vi "Pixy_COM-RIO.vi"() -> (0 "Height":i32, 1 "Width":i32, 2 "Y":i32, 3 "X":i32, 4 "Read error out":errorcluster)   [LabVIEW 2016]
uses:
  <vilib>/Analysis/baseanly.llb/Mean (DBL).vi
  <vilib>/Instr/_visa.llb/VISA Configure Serial Port (Instr).vi
  Cam Area.vi
  Cam H.vi
  Cam W.vi
  Cam Y.vi
  Cam X.vi
  <vilib>/Analysis/NI_AALBase.lvlib
panel:
  in  "Command 2":string(combo)="go"
  out "Initialization error out":errorcluster
  out "Area":dbl(graph)
  in  "Display buffer size":u16=100 min=1
  out "Data display":string
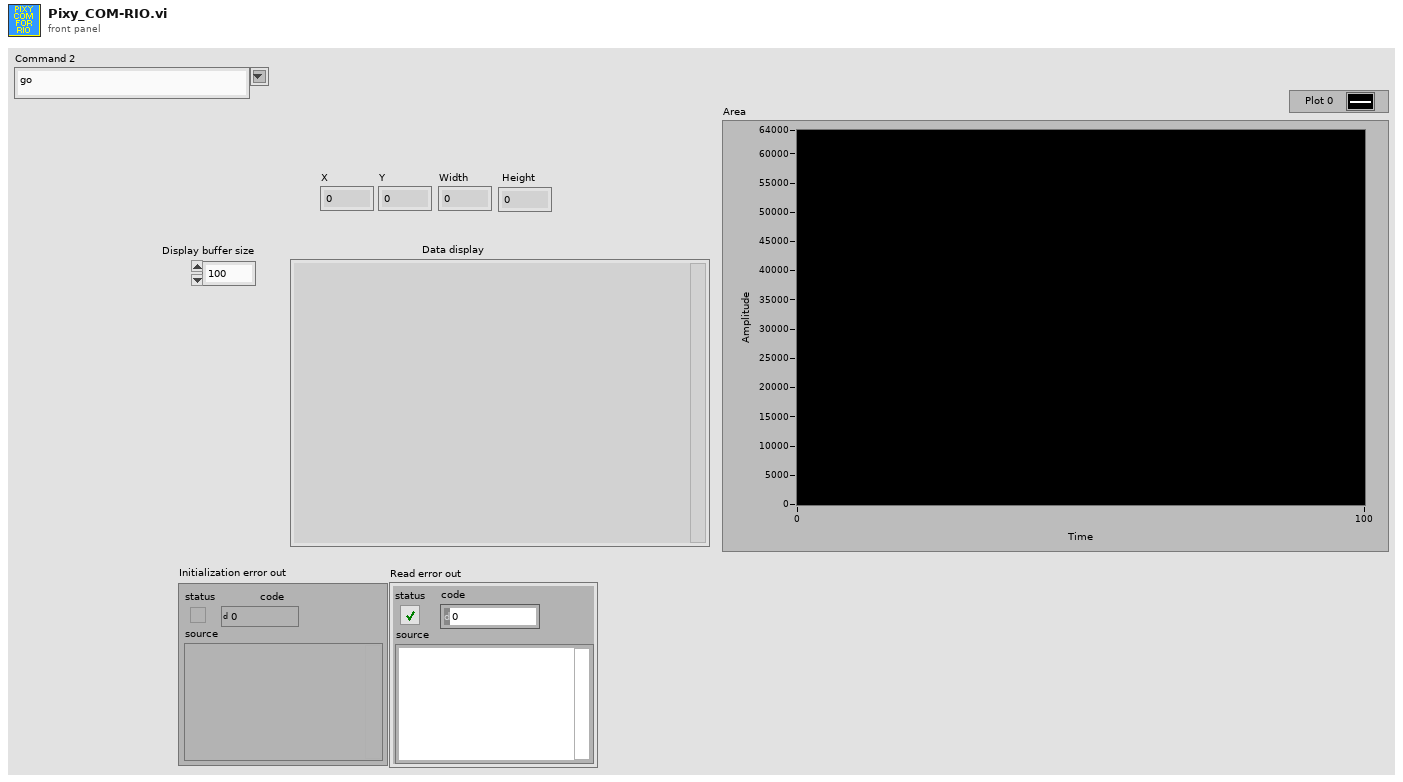
[diagram p1: front panel]
types:
  T1 = cluster{"buffer":string, "X":i32, "Y":i32, "Width":i32, "Height":i32, "Area":dbl}
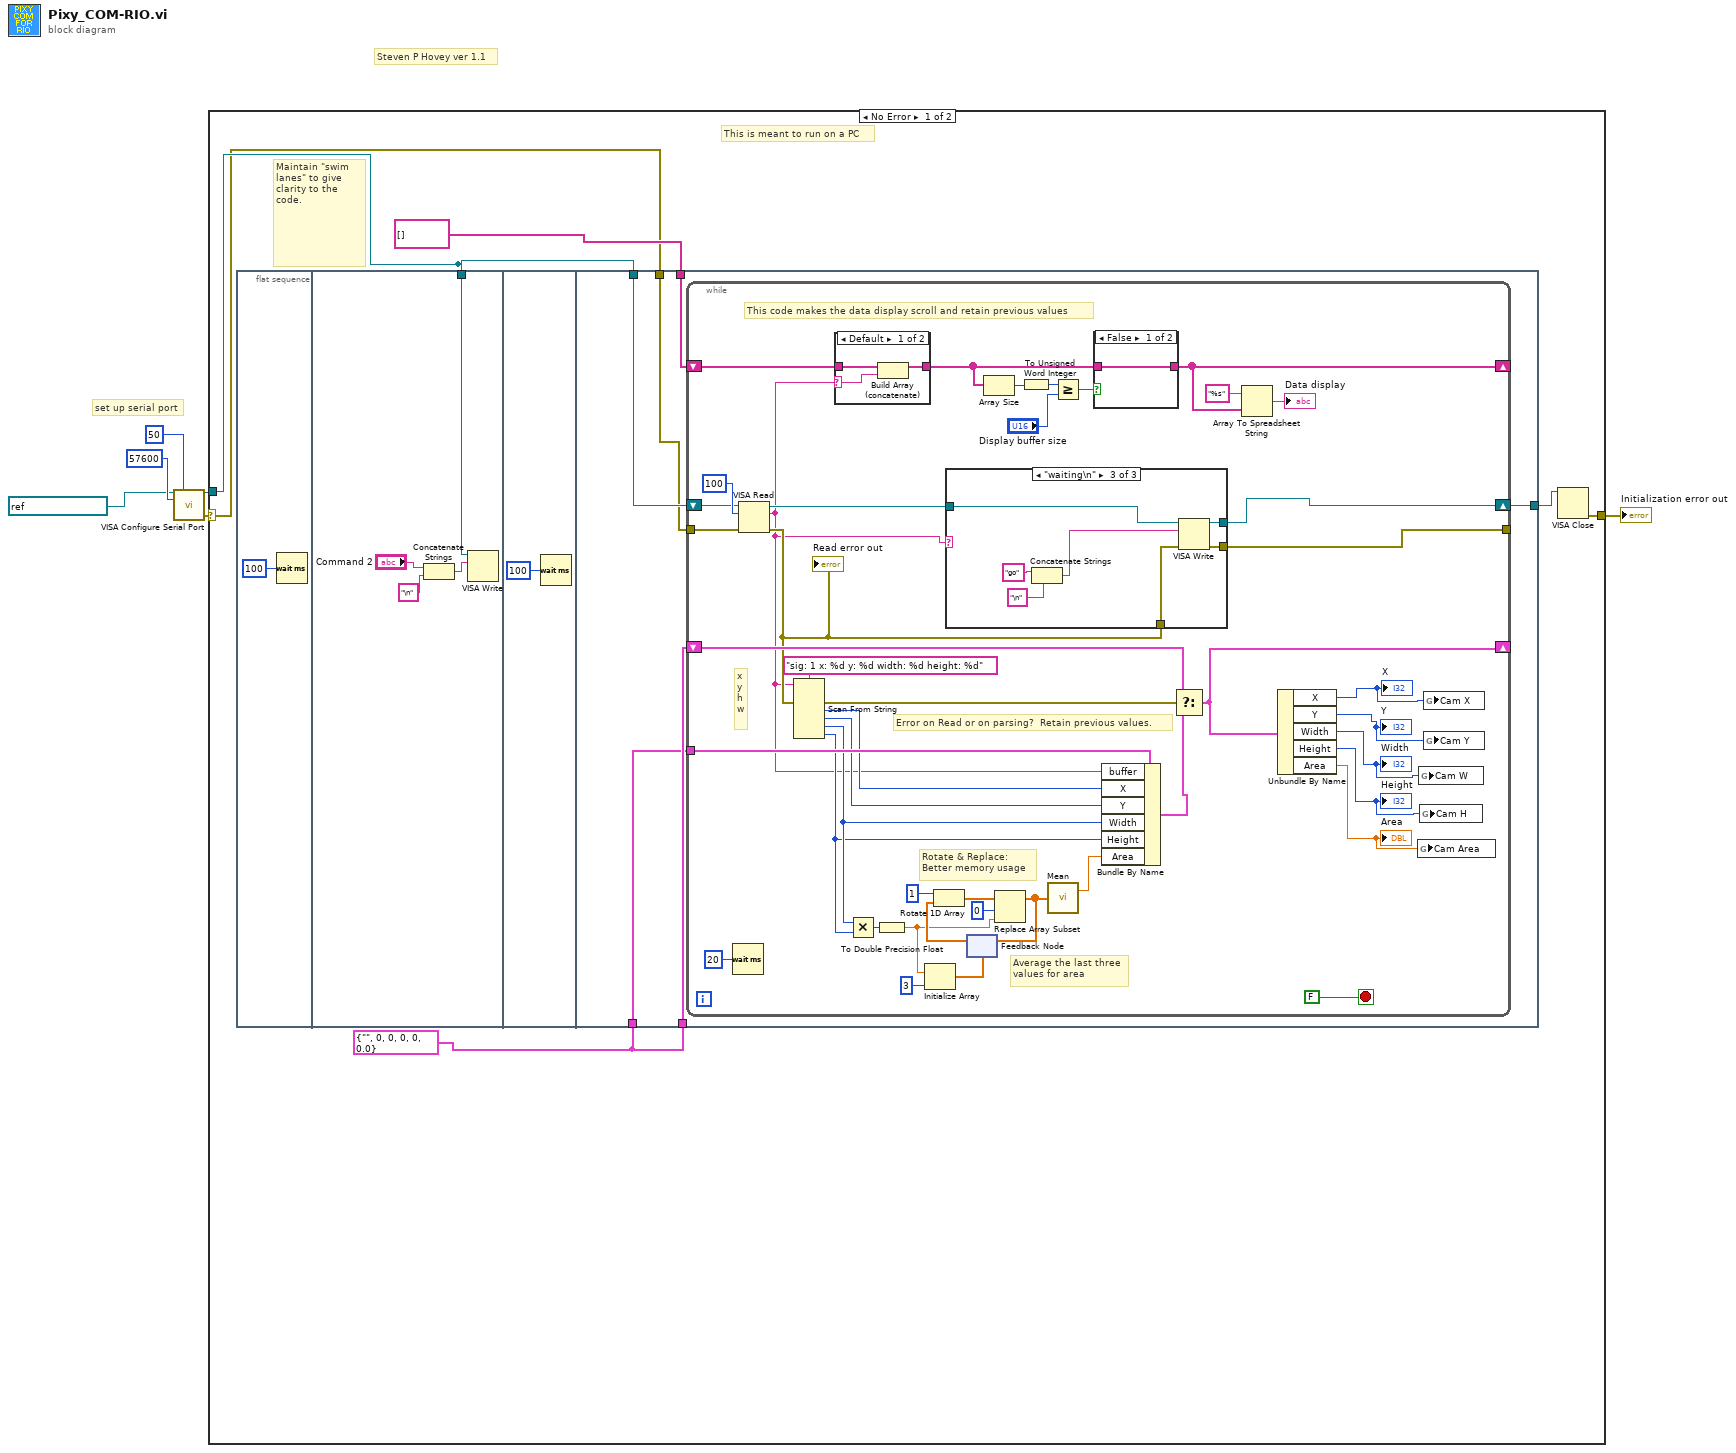
[diagram p0: block diagram]
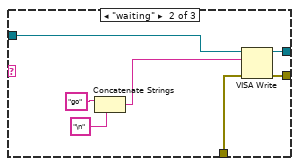
[diagram p3: hidden frame]
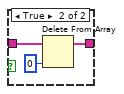
[diagram p5: hidden frame]
diagram:
  # "Steven P Hovey ver 1.1"
  # "set up serial port"
  n1 = call-poly "VISA Configure Serial Port"("VISA resource name"=refnum<visa-resource-name> "ASRL3::INSTR", "timeout (10sec)"=u32 50, "baud rate (9600)"=u32 57600) -> ("VISA resource name out"=w4:refnum<visa-resource-name>, "error out"=w2:errorcluster)  [unwired: 11 in]
  n2 = case shown="No Error" w2 {
    selector: w2 -> [w8 w93]
    tunnel: w4 -> [w9 _]
    tunnel: [w12 w93] -> w3
    frame No Error {
      w10 = T1 {"buffer"="", "X"=0, "Y"=0, "Width"=0, "Height"=0, "Area"=0.0}
      # "Maintain \"swim lanes\" to give clarity to the code."
      # "This is meant to run on a PC"
      n3 = flat-sequence {
        tunnel: w9 -> [w15]
        tunnel: string[] [] -> [w24]
        tunnel: w10 -> [w23]
        tunnel: w10 -> [w22]
        tunnel: w9 -> [w21]
        tunnel: w8 -> [w20]
        tunnel: [w19] -> w7
        frame #0 {
          n4 = Wait (ms)(milliseconds to wait=u32 100) -> ()  [unwired: 1 out]
        }
        frame #1 {
          n5 = Concatenate Strings("Command 2", "\n") -> (w17:string)
          n6 = VISA Write(VISA resource name=w15, write buffer=w17) -> ()  [unwired: 1 in, 3 out]
        }
        frame #2 {
          n7 = Wait (ms)(milliseconds to wait=u32 100) -> ()  [unwired: 1 out]
        }
        frame #3 {
          n8 = while {
            shift-right: [w28] -> w19
            shift-left: w21 -> [w65]
            shift-right: [w44] -> _
            shift-left: w23 -> [w45]
            shift-right: [w38] -> _
            shift-left: w24 -> [w58]
            tunnel: w22 -> [w68]
            tunnel: w20 -> [w37]
            tunnel: [w27] -> _
            stop <- FALSE ("stop") stop-if-true
            # "Error on Read or on parsing?  Retain previous values."
            # "Rotate & Replace:\nBetter memory usage"
            # "Average the last three\nvalues for area"
            # "This code makes the data display scroll and retain previous values"
            # "x\ny\nh\nw"
            n9 = Wait (ms)(milliseconds to wait=u32 20) -> ()  [unwired: 1 out]
            n10 = VISA Read(VISA resource name=w65, byte count=u32 100, error in (no error)=w37) -> (VISA resource name out=w29:refnum<visa-resource-name>, read buffer=w25:string, error out=w26:errorcluster)  [unwired: 1 out]
            "Read error out" <- w26
            n11 = Scan From String(format string="sig: 1 x: %d y: %d width: %d height: %d", input string=w25, error in=w26) -> (error out=w46:errorcluster, output 1=w51:i32, output 2=w50:i32, output 3=w49:i32, output 4=w48:i32)  [unwired: 5 in, 2 out]
            n12 = case shown="Default" w25 {
              selector: w25 -> [w85 _]
              tunnel: w58 -> [w86 w88]
              tunnel: [w87 w88] -> w39
              frame Default {
                n13 = Build Array (concatenate)(w86, w85) -> (w87:string[])
              }
              frame "" {
              }
            }
            n14 = Multiply(x=w49, y=w48) -> (x*y=w47:i32)
            n15 = To Double Precision Float(number=w47) -> (double precision float=w40:dbl)
            n16 = Initialize Array(w40, 3 ("dimension size")) -> (w62:dbl[])
            n17 = case shown="\"waiting\\n\"" w25 {
              tunnel: w29 -> [w70 w77 w84]
              tunnel: [w70 w76 w83] -> w28
              tunnel: [w69 w75 w82] -> w27
              tunnel: w26 -> [w69 w72 w79]
              frame "False", Default {
              }
              frame "waiting" {
                n18 = Concatenate Strings("go", "\n") -> (w71:string)
                n19 = VISA Write(VISA resource name=w77, write buffer=w71, error in (no error)=w72) -> (VISA resource name out=w76:refnum<visa-resource-name>, error out=w75:errorcluster)  [unwired: 1 out]
              }
              frame "waiting\n" {
                n20 = Concatenate Strings("go", "\n") -> (w78:string)
                n21 = VISA Write(VISA resource name=w84, write buffer=w78, error in (no error)=w79) -> (VISA resource name out=w83:refnum<visa-resource-name>, error out=w82:errorcluster)  [unwired: 1 out]
              }
            }
            n22 = feedback #1(w62) -> (w43:dbl[])
            n23 = Rotate 1D Array(1:w43, 2:1 ("n")) -> (0:w42:dbl[])
            n24 = Array Size(array=w39) -> (size(s)=w56:i32)
            n25 = Replace Array Subset(array=w42, new element=w40, index=0) -> (w61:dbl[])
            n26 = feedback-in #1(w61) -> ()
            n27 = To Unsigned Word Integer(number=w56) -> (unsigned 16bit integer=w55:u16)
            n28 = call-poly <vilib>:"Mean.vi"("X"=w61) -> ("mean"=w64:dbl)  [unwired: 1 out]
            n29 = Greater Or Equal?(x=w55, y="Display buffer size") -> (x >= y?=w54:bool)
            n30 = case shown="False" w54 {
              tunnel: w39 -> [w89 w92]
              tunnel: [w89 w91] -> w38
              frame False {
              }
              frame True {
                n31 = Delete From Array(array=w92, index=0) -> (array with subset deleted=w91:string[])  [unwired: 1 in, 1 out]
              }
            }
            n32 = Bundle By Name(cluster=w68, "buffer"=w25, "X"=w51, "Y"=w50, "Width"=w49, "Height"=w48, "Area"=w64) -> (w30:T1)
            n33 = Select(t=w45, s=w46, f=w30) -> (s? t:f=w44:T1)
            n34 = Array To Spreadsheet String(array=w38, 3:"%s" ("format string")) -> (spreadsheet string=→"Data display":string)  [unwired: 1 in]
            n35 = Unbundle By Name(w44) -> ("X"=w33:i32, "Y"=w32:i32, "Width"=w35:i32, "Height"=w34:i32, "Area"=w31:dbl)
            "X" <- w33
            "Y" <- w32
            "Width" <- w35
            "Height" <- w34
            "Area" <- w31
            n36 = global write "Cam Area.vi" "Cam Area"(w31) -> ()
            n37 = global write "Cam W.vi" "Cam W"(w35) -> ()
            n38 = global write "Cam H.vi" "Cam H"(w34) -> ()
            n39 = global write "Cam X.vi" "Cam X"(w33) -> ()
            n40 = global write "Cam Y.vi" "Cam Y"(w32) -> ()
          }
        }
      }
      n41 = VISA Close(VISA resource name=w7) -> (error out=w12:errorcluster)  [unwired: 1 in]
    }
    frame Error {
    }
  }
  "Initialization error out" <- w3
